vi "MB Ethernet Slave Demon.vi"(9 "Period":u32=75, 10 "Timeout":i32=5000, 11 "Port":u16=502) -> (2 "Demon Running":bool, 3 "# of connections":i32)   [LabVIEW 2013]
doc: "The Ethernet slave demon waits and establishes connection to Ethernet masters. It then constantly scans the TCP buffer for commands from the master. When it detects a command from the master, it updates the memory tables with data and also responds to the master's query for data. You must use the Slave API to access the data in the tables."
uses:
  NI Modbus.llb/MB Ethernet Connection Function.ctl
  NI Modbus.llb/MB RefCount Function.ctl
  NI Modbus.llb/MB Globals.vi
panel:
  in  "Case Constant\n(See Context Help)":bool
  # "VI Name: MB Ethernet Slave Demon.vi\nPurpose: Modbus Demon\nMonitor a single port, but can accept multiple connections."
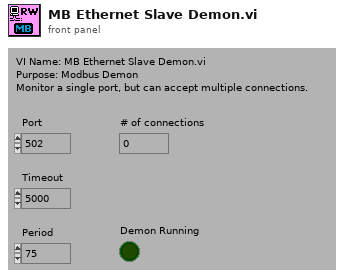
[diagram p1: front panel]
types:
  T1 = typedef "MB RefCount Function.ctl" = enum16{"Init", "Add", "Remove", "Is Running?"}
  T2 = typedef "MB Ethernet Connection Function.ctl" = enum16{"Init", "Add Connection", "Get All Connections", "Delete Connection"}
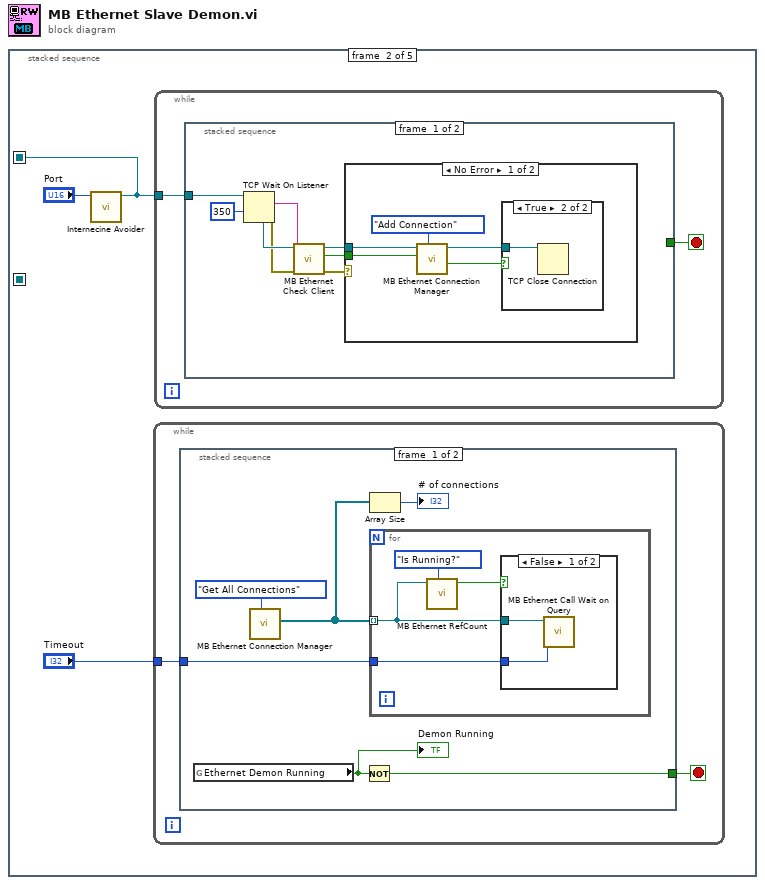
[diagram p0: block diagram]
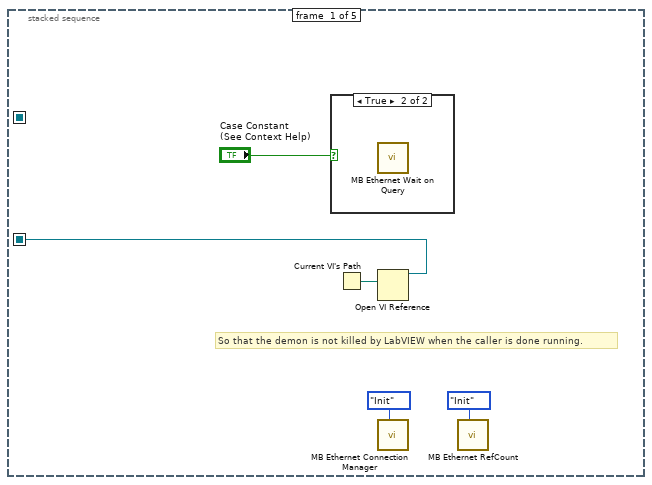
[diagram p2: hidden frame]
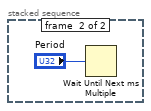
[diagram p5: hidden frame]
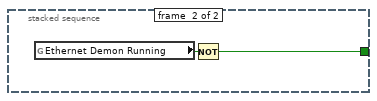
[diagram p8: hidden frame]
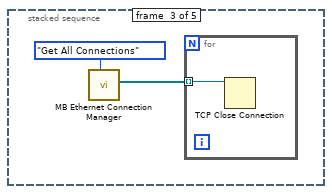
[diagram p9: hidden frame]
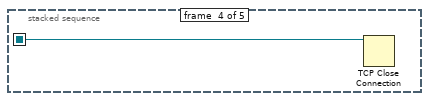
[diagram p10: hidden frame]
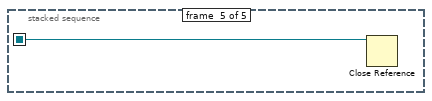
[diagram p11: hidden frame]
diagram:
  n1 = stacked-sequence {
    seq-local: [w4 _ _ _ _] -> [_ _ _ _ w46]
    seq-local: [_ w6 _ _ _] -> [_ _ _ w45 _]
    frame #0 {
      # "So that the demon is not killed by LabVIEW when the caller is done running."
      n2 = case shown="True" "Case Constant\n(See Context Help)" {
        frame False {
        }
        frame True {
          n3 = call "MB Ethernet Wait on Query.vi"() -> ()  [unwired: 2 in, 10 out]
        }
      }
      n4 = Current VI's Path() -> (path=w5:path)
      n5 = Open VI Reference(vi path=w5) -> (vi reference=w4:refnum<vi>)  [unwired: 1 in, 5 out]
      n6 = call "MB Ethernet Connection Manager.vi"("Function"=MB_Ethernet_Connection_Function."Init") -> ()  [unwired: 2 in, 9 out]
      n7 = call "MB Ethernet RefCount.vi"("Function"=MB_RefCount_Function."Init") -> ()  [unwired: 1 in, 10 out]
    }
    frame #1 {
      n8 = call <vilib>:"Internecine Avoider.vi"("port"="Port") -> ("connection ID"=w6:refnum<k5>)  [unwired: 3 in, 7 out]
      n9 = while {
        tunnel: "Timeout" -> [w9]
        stop <- w10 stop-if-true
        n10 = stacked-sequence {
          tunnel: [w16 _] -> w10
          tunnel: w9 -> [w11 _]
          frame #0 {
            n11 = global read "MB Globals.vi" "Ethernet Demon Running"() -> (w15:bool)
            "Demon Running" <- w15
            n12 = call "MB Ethernet Connection Manager.vi"("Function"=MB_Ethernet_Connection_Function."Get All Connections") -> ("Connection IDs"=w12:refnum<k5>[])  [unwired: 2 in, 8 out]
            n13 = Not(x=w15) -> (.not. x?=w16:bool)
            n14 = Array Size(array=w12) -> (size(s)=→"# of connections":i32)
            n15 = for {
              tunnel: w12 -> [w18] mode=indexing
              tunnel: w11 -> [w19]
              n16 = call "MB Ethernet RefCount.vi"("Function"=MB_RefCount_Function."Is Running?", "Connection ID"=w18) -> ("VI Running?"=w17:bool)  [unwired: 9 out]
              n17 = case shown="False" w17 {
                tunnel: w18 -> [w22 _]
                tunnel: w19 -> [w21 _]
                frame False {
                  n18 = call "MB Ethernet Call Wait on Query.vi"("Timeout"=w21, "Connection ID"=w22) -> ()  [unwired: 10 out]
                }
                frame True {
                }
              }
            }
          }
          frame #1 {
            n19 = Wait Until Next ms Multiple(millisecond multiple="Period") -> ()  [unwired: 1 out]
          }
        }
      }
      n20 = while {
        tunnel: w6 -> [w25]
        stop <- w24 stop-if-true
        n21 = stacked-sequence {
          tunnel: w25 -> [w33 _]
          tunnel: [_ w40] -> w24
          frame #0 {
            n22 = TCP Wait On Listener(9:350 ("timeout ms (wait forever: -1)"), 11:w33) -> (0:w30:errorcluster, 2:w28:string, 4:w32:refnum<k5>)  [unwired: 1 in, 3 out]
            n23 = call "MB Ethernet Check Client.vi"("error in (no error)"=w30, "Remote Address"=w28, "Connection ID in"=w32) -> ("error out"=w29:errorcluster, "Priority"=w27:bool, "Connection ID out"=w31:refnum<k5>)  [unwired: 6 out]
            n24 = case shown="No Error" w29 {
              tunnel: w31 -> [w38 _]
              tunnel: w27 -> [w34 _]
              frame No Error {
                n25 = call "MB Ethernet Connection Manager.vi"("Function"=MB_Ethernet_Connection_Function."Add Connection", "Priority"=w34, "Connection ID"=w38) -> ("Close Connection"=w36:bool, "Connection ID to Delete"=w35:refnum<k5>)  [unwired: 7 out]
                n26 = case shown="True" w36 {
                  tunnel: w35 -> [_ w39]
                  frame False {
                  }
                  frame True {
                    n27 = TCP Close Connection(connection ID=w39) -> ()  [unwired: 1 in, 3 out]
                  }
                }
              }
              frame Error {
              }
            }
          }
          frame #1 {
            n28 = global read "MB Globals.vi" "Ethernet Demon Running"() -> (w41:bool)
            n29 = Not(x=w41) -> (.not. x?=w40:bool)
          }
        }
      }
    }
    frame #2 {
      n30 = call "MB Ethernet Connection Manager.vi"("Function"=MB_Ethernet_Connection_Function."Get All Connections") -> ("Connection IDs"=w42:refnum<k5>[])  [unwired: 2 in, 8 out]
      n31 = for {
        tunnel: w42 -> [w44] mode=indexing
        n32 = TCP Close Connection(connection ID=w44) -> ()  [unwired: 1 in, 3 out]
      }
    }
    frame #3 {
      n33 = TCP Close Connection(connection ID=w45) -> ()  [unwired: 1 in, 3 out]
    }
    frame #4 {
      n34 = Close Reference(reference=w46) -> ()  [unwired: 1 in, 1 out]
    }
  }
